vi "Pedestrian Signal Controller (Walk).vi"(11 "cars stopped":T1) -> (0 "ped signal":T2, 3 "peds stopped":T1)   [LabVIEW 2023]
uses:
  <extravilib>/ChannelInstances/One Element Stream-u16/)Channel.ctl
  <extravilib>/ChannelInstances/One Element Stream-bool/)Channel.ctl
  e765195b-037f-ea4a-882a-d3299082ef25.vi
  091f0f9f-ba83-5e49-bf52-7e477d967a4d.vi
  <extravilib>/ChannelInstances/One Element Stream-u16/Write With Abort.vi
  <extravilib>/ChannelInstances/One Element Stream-bool/Write With Abort.vi
  <extravilib>/ChannelInstances/One Element Stream-bool/Read With Abort.vi
  <extravilib>/ChannelInstances/One Element Stream-u16/Endpoint.vi
  <extravilib>/ChannelInstances/One Element Stream-bool/Endpoint.vi
  <extravilib>/ChannelInstances/One Element Stream-bool/EndpointRead.vi
  <extravilib>/ChannelInstances/One Element Stream-bool.lvlib
  <extravilib>/ChannelInstances/One Element Stream-u16.lvlib
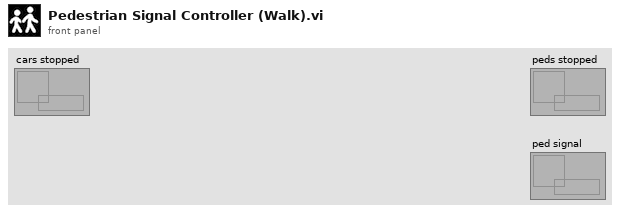
[diagram p1: front panel]
types:
  T1 = typedef "One Element Stream-bool.lvlib/)Channel.ctl" = refnum<queue>
  T2 = typedef "One Element Stream-u16.lvlib/)Channel.ctl" = refnum<queue>
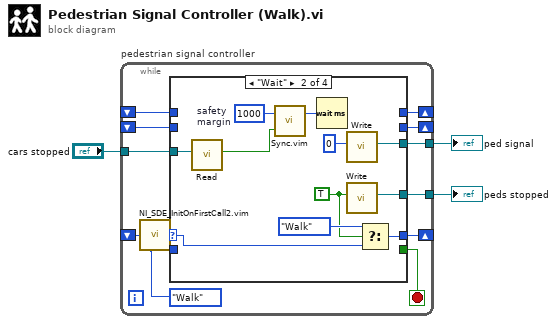
[diagram p0: block diagram]
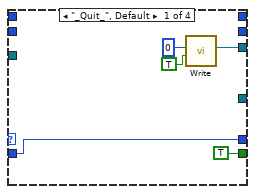
[diagram p2: hidden frame]
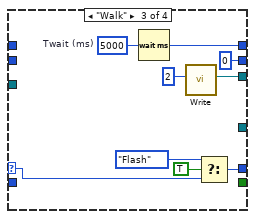
[diagram p3: hidden frame]
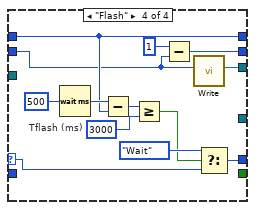
[diagram p4: hidden frame]
diagram:
  n1 = while "pedestrian signal controller" {
    tunnel: "cars stopped" -> [w14]
    shift-right: [w13] -> _
    shift-left: _ -> [w12]
    tunnel: [w11] -> w3
    shift-right: [w10] -> _
    shift-left: _ -> [w9]
    tunnel: [w8] -> w2
    shift-right: [w6] -> _
    shift-left: _ -> [w5]
    stop <- w15 stop-if-true
    w7 = enum16{"_Quit_", "Wait", "Walk", "Flash"}."Walk"
    n2 = call "NI_SDE_InitOnFirstCall2.vim"("input"=w5, "master enum"=w7) -> ("output enum"=w4:enum16{"_Quit_", "Wait", "Walk", "Flash"})  [unwired: 1 in]
    n3 = case shown="\"Wait\"" w4 {
      selector: w4 -> [_ w31 w40 w53]
      tunnel: [TRUE _ _ _] -> w15
      tunnel: [w16 w30 w39 w52] -> w6
      tunnel: w14 -> [_ w28 _ _]
      tunnel: [_ _ w35 w46] -> w13
      tunnel: w12 -> [_ _ _ w46]
      tunnel: [w18 w26 w33 w45] -> w11
      tunnel: [_ _ u16 0 w43] -> w10
      tunnel: w9 -> [_ _ _ w42]
      tunnel: [_ w25 _ _] -> w8
      tunnel: w7 -> [w16 _ _ _]
      frame "_Quit_", Default {
        n4 = call <extravilib>:"Write.vi"("last element? (F)"=TRUE, "element"=u16 0) -> ("channel"=w18:T2)  [unwired: 8 in, 1 out]
      }
      frame "Wait" {
        w21 = TRUE
        w23 = u32 1000  # safety margin
        n5 = call <extravilib>:"Read.vi"("channel"=w28) -> ("element"=w24:bool)  [unwired: 7 in, 3 out]
        n6 = call "Sync.vim"("a"=w23, "b"=w24) -> ("a'"=w22:u32)  [unwired: 24 in, 1 out]
        n7 = Wait (ms)(milliseconds to wait=w22) -> ()  [unwired: 1 out]
        n8 = call <extravilib>:"Write.vi"("element"=u16 0) -> ("channel"=w26:T2)  [unwired: 9 in, 1 out]
        n9 = call <extravilib>:"Write.vi"("element"=w21) -> ("channel"=w25:T1)  [unwired: 9 in, 1 out]
        n10 = Select(t=enum16{"_Quit_", "Wait", "Walk", "Flash"}."Walk", s=w21, f=w31) -> (s? t:f=w30:enum16{"_Quit_", "Wait", "Walk", "Flash"})
      }
      frame "Walk" {
        w37 = u32 5000  # Twait (ms)
        n11 = Wait (ms)(milliseconds to wait=w37) -> (millisecond timer value=w35:u32)
        n12 = call <extravilib>:"Write.vi"("element"=u16 2) -> ("channel"=w33:T2)  [unwired: 9 in, 1 out]
        n13 = Select(t=enum16{"_Quit_", "Wait", "Walk", "Flash"}."Flash", s=TRUE, f=w40) -> (s? t:f=w39:enum16{"_Quit_", "Wait", "Walk", "Flash"})
      }
      frame "Flash" {
        w47 = u32 3000  # Tflash (ms)
        n14 = Wait (ms)(milliseconds to wait=u32 500) -> (millisecond timer value=w49:u32)
        n15 = Subtract(x=w49, y=w46) -> (x-y=w48:u32)
        n16 = Greater Or Equal?(x=w48, y=w47) -> (x >= y?=w41:bool)
        n17 = Subtract(x=u16 1, y=w42) -> (x-y=w43:u16)
        n18 = call <extravilib>:"Write.vi"("element"=w42) -> ("channel"=w45:T2)  [unwired: 9 in, 1 out]
        n19 = Select(t=enum16{"_Quit_", "Wait", "Walk", "Flash"}."Wait", s=w41, f=w53) -> (s? t:f=w52:enum16{"_Quit_", "Wait", "Walk", "Flash"})
      }
    }
  }
  "ped signal" <- w3
  "peds stopped" <- w2
